vi "tcp_server_monitor.vi"(11 "TCP Socket Server in":refnum<data-value>) -> ()   [LabVIEW 2019, in "TCP Socket Server.lvclass"]
uses:
  TCP Socket Server.lvclass
  TCP Socket Server.lvclass/TCP Socket Server.ctl
  Utility API/Log Service/public/level.ctl
  df063e67-b3ba-41cf-b203-ca072a03e9e6.vi
  6658b09d-3cc9-4502-9e9e-f034e714faf1.vi
  e82c1857-569d-4e52-8d07-6a4305579ab7.vi
  Util/Timestamp or now.vi
  TCP Connection/TCP Connection.lvclass
  C:/Users/Nicholas Folse/Documents/workspace/github-tauterra.llc/ANODE/ANODE/Socket API/Connection/Connection.lvclass
  Socket Server/subVIs/spawn_connection_handler.vi
  Utility API/Log Service/Log Service.lvclass
  Socket Server/Socket Server.lvclass
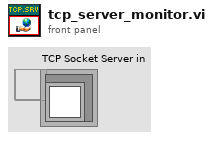
[diagram p1: front panel]
types:
  T1 = typedef "Utility API.lvlib/Log Service.lvclass/level.ctl" = u16
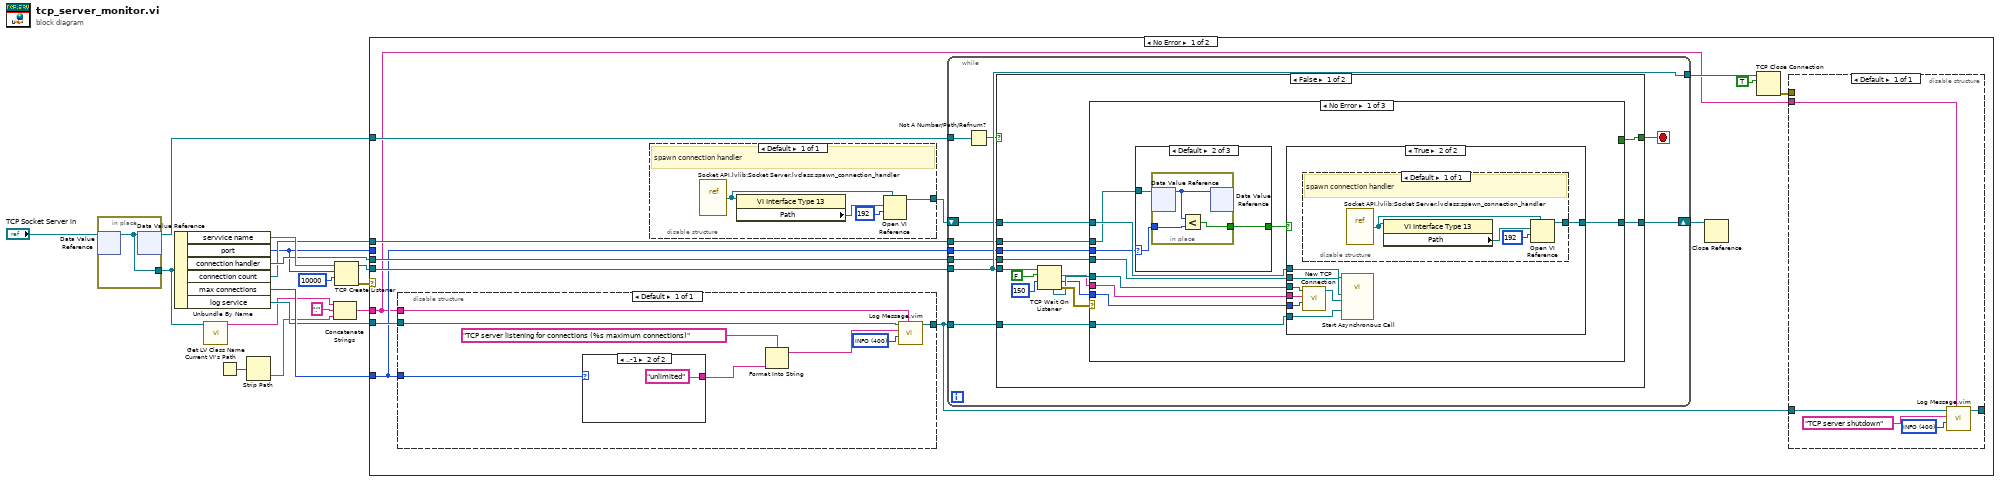
[diagram p0: block diagram]
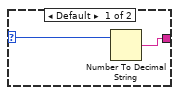
[diagram p2: hidden frame]
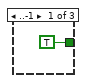
[diagram p3: hidden frame]
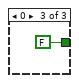
[diagram p4: hidden frame]
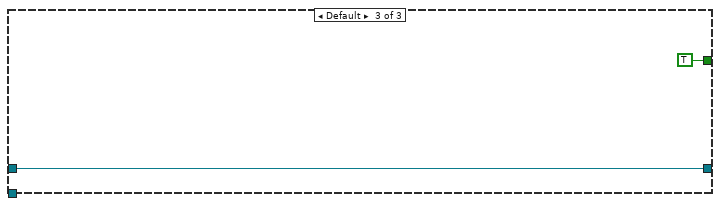
[diagram p7: hidden frame]
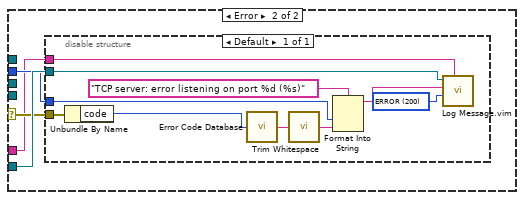
[diagram p9: hidden frame]
diagram:
  n1 = in-place {
    in-place-border: [w18] -> w5
    n2 = in-place-dvr #1("TCP Socket Server in") -> (w18:refnum<class "TCP Socket Server.lvclass">)  [unwired: 1 out]
    n3 = in-place-dvr #1(w18) -> (w11:refnum<data-value>)  [unwired: 1 out]
  }
  n4 = Unbundle By Name(w5) -> ("servvice name"=w16:string, "port"=w6:u16, "connection handler"=w12:refnum<class "Connection Handler.lvclass">, "connection count"=w10:refnum<data-value>, "max connections"=w9:i32, "log service"=w8:refnum<data-value>)
  n5 = call <vilib>:"Get LV Class Name.vi"("object"=w5) -> ("class name"=w3:string)  [unwired: 9 in, 1 out]
  n6 = Current VI's Path() -> (path=w7:path)
  n7 = Strip Path(path=w7) -> (name=w2:string)  [unwired: 1 out]
  n8 = Concatenate Strings(w3, ":" ("string"), w2) -> (w1:string)
  n9 = TCP Create Listener(9:10000 ("timeout ms (25000)"), 10:w6, 11:w16) -> (0:w14:errorcluster, 3:w13:refnum<k5>)  [unwired: 2 in, 1 out]
  n10 = case shown="No Error" w14 {
    selector: w14 -> [_ w114]
    tunnel: w13 -> [w31 _]
    tunnel: w11 -> [w30 _]
    tunnel: w12 -> [w27 _]
    tunnel: w10 -> [w24 _]
    tunnel: w9 -> [w22 _]
    tunnel: w8 -> [w23 w115]
    tunnel: w1 -> [w19 w112]
    tunnel: w6 -> [_ w113]
    frame No Error {
      n11 = disable-structure shown="Default" {
        disable-tunnel: w23 -> [w44]
        disable-tunnel: w22 -> [w43]
        disable-tunnel: w19 -> [w41]
        disable-tunnel: [w37] -> w20
        frame Enabled {
          w42 = T1 400 items=["OFF"=0, "FATAL"=100, "ERROR"=200, "WARN"=300, "INFO"=400, "DEBUG"=500, "TRACE"=600, "ALL"=65535] ("level")
          n12 = case shown="..-1" w43 {
            selector: w43 -> [w46 _]
            tunnel: [w45 "unlimited"] -> w39
            frame Default {
              n13 = Number To Decimal String(number=w46) -> (decimal integer string=w45:string)  [unwired: 1 in]
            }
            frame ..-1 {
            }
          }
          n14 = Format Into String(format string="TCP server listening for connections (%s maximum connections)" ("message"), w39) -> (resulting string=w38:string)  [unwired: 2 in, 1 out]
          n15 = call "Log Message.vim"("context"=w41, "level"=w42, "message"=w38, "Log Service in"=w44) -> ("Log Service out"=w37:refnum<data-value>)  [unwired: 6 in, 1 out]
        }
      }
      n16 = disable-structure shown="Default" {
        disable-tunnel: [w48] -> w26
        frame Enabled {
          # "spawn connection handler"
          n17 = vi-ref "Socket API.lvlib:Socket Server.lvclass:spawn_connection_handler.vi"() -> (w49:refnum<vi>)
          n18 = property class="VI Interface Type 13"(reference=w49) -> ("Path"=w50:path)  [unwired: 1 in, 2 out]
          n19 = Open VI Reference(type specifier VI Refnum (for type only)=w49, vi path=w50, options=192) -> (vi reference=w48:refnum<vi>)  [unwired: 3 in, 1 out]
        }
      }
      n20 = while {
        tunnel: w31 -> [w61]
        tunnel: w30 -> [w59]
        tunnel: [w61] -> w29
        tunnel: w27 -> [w60]
        shift-right: [w55] -> w25
        shift-left: w26 -> [w56]
        tunnel: w24 -> [w54]
        tunnel: w22 -> [w53]
        tunnel: w20 -> [w52]
        stop <- w57 stop-if-true
        n21 = Not A Number/Path/Refnum?(number/path/refnum=w59) -> (NaN/Path/Refnum?=w58:bool)
        n22 = case shown="False" w58 {
          selector: w58 -> [_ w111]
          tunnel: [w70 w111] -> w57
          tunnel: w61 -> [w75 _]
          tunnel: w60 -> [w67 _]
          tunnel: w56 -> [w66 w110]
          tunnel: [w65 w110] -> w55
          tunnel: w54 -> [w64 _]
          tunnel: w53 -> [w63 _]
          tunnel: w52 -> [w62 _]
          frame False {
            n23 = TCP Wait On Listener(9:150 ("timeout ms (wait forever: -1)"), 10:FALSE ("resolve remote address (T)"), 11:w75) -> (0:w72:errorcluster, 1:w68:u16, 2:w69:string, 4:w71:refnum<k5>)  [unwired: 1 in, 1 out]
            n24 = case shown="No Error" w72 {
              tunnel: w71 -> [w85 _ _]
              tunnel: [_ _ TRUE] -> w70
              tunnel: w69 -> [w84 _ _]
              tunnel: w68 -> [w83 _ _]
              tunnel: w67 -> [w82 _ _]
              tunnel: w66 -> [w81 w107 w108]
              tunnel: [w80 w107 w108] -> w65
              tunnel: w64 -> [w79 _ _]
              tunnel: w63 -> [w77 _ _]
              tunnel: w62 -> [w76 _ _]
              frame No Error {
                n25 = case shown="Default" w77 {
                  selector: w77 -> [_ w87 _]
                  tunnel: w79 -> [_ w89 _]
                  tunnel: [TRUE w88 FALSE] -> w78
                  frame ..-1 {
                  }
                  frame Default {
                    n26 = in-place {
                      in-place-border: w87 -> [w92]
                      in-place-border: [w90] -> w88
                      n27 = in-place-dvr #2(w89) -> (w91:i32)  [unwired: 1 out]
                      n28 = Less?(x=w91, y=w92) -> (x < y?=w90:bool)
                      n29 = in-place-dvr #2(w91) -> ()  [unwired: 2 out]
                    }
                  }
                  frame 0 {
                  }
                }
                n30 = case shown="True" w78 {
                  tunnel: w85 -> [_ w102]
                  tunnel: w84 -> [_ w101]
                  tunnel: w83 -> [_ w100]
                  tunnel: w82 -> [_ w99]
                  tunnel: w81 -> [w94 w97]
                  tunnel: [w94 w96] -> w80
                  tunnel: w76 -> [_ w95]
                  frame False {
                  }
                  frame True {
                    n31 = disable-structure shown="Default" {
                      disable-tunnel: [w103] -> w96
                      frame Enabled {
                        # "spawn connection handler"
                        n32 = vi-ref "Socket API.lvlib:Socket Server.lvclass:spawn_connection_handler.vi"() -> (w104:refnum<vi>)
                        n33 = property class="VI Interface Type 13"(reference=w104) -> ("Path"=w105:path)  [unwired: 1 in, 2 out]
                        n34 = Open VI Reference(type specifier VI Refnum (for type only)=w104, vi path=w105, options=192) -> (vi reference=w103:refnum<vi>)  [unwired: 3 in, 1 out]
                      }
                    }
                    n35 = call "New TCP Connection.vi"("remote port"=w100, "remote address"=w101, "connection ID"=w102) -> ("TCP Connection out"=w98:refnum<class "TCP Connection.lvclass">)  [unwired: 7 in, 1 out]
                    n36 = call-by-ref "Start Asynchronous Call"(reference=w97, "Log Service"=w95, "Connection"=w98, "Connection Hanlder"=w99) -> ()  [unwired: 10 in, 2 out]
                  }
                }
              }
              frame Error {
                # "timeout"
              }
              frame Default {
              }
            }
          }
          frame True {
          }
        }
      }
      n37 = Close Reference(reference=w25) -> ()  [unwired: 1 in, 1 out]
      n38 = TCP Close Connection(connection ID=w29, abort (F)=TRUE) -> (error out=w21:errorcluster)  [unwired: 1 in, 1 out]
      n39 = disable-structure shown="Default" {
        disable-tunnel: w20 -> [w36]
        disable-tunnel: w19 -> [w34]
        disable-tunnel: [w33] -> _
        disable-tunnel: w21 -> [_]
        frame Enabled {
          w35 = T1 400 items=["OFF"=0, "FATAL"=100, "ERROR"=200, "WARN"=300, "INFO"=400, "DEBUG"=500, "TRACE"=600, "ALL"=65535] ("level")
          n40 = call "Log Message.vim"("context"=w34, "level"=w35, "message"="TCP server shutdown", "Log Service in"=w36) -> ("Log Service out"=w33:refnum<data-value>)  [unwired: 6 in, 1 out]
        }
      }
    }
    frame Error {
      n41 = disable-structure shown="Default" {
        disable-tunnel: w115 -> [w125]
        disable-tunnel: w114 -> [w123]
        disable-tunnel: w113 -> [w120]
        disable-tunnel: w112 -> [w116]
        frame Enabled {
          w124 = T1 200 items=["OFF"=0, "FATAL"=100, "ERROR"=200, "WARN"=300, "INFO"=400, "DEBUG"=500, "TRACE"=600, "ALL"=65535] ("level")
          n42 = Unbundle By Name(w123) -> ("code"=w122:i32)
          n43 = call <vilib>:"Error Code Database.vi"("Error Code"=w122) -> ("Error Text"=w119:string)
          n44 = call <vilib>:"Trim Whitespace.vi"("string"=w119) -> ("trimmed string"=w118:string)  [unwired: 1 in]
          n45 = Format Into String(format string="TCP server: error listening on port %d (%s)" ("message"), w120, w118) -> (resulting string=w117:string)  [unwired: 2 in, 1 out]
          n46 = call "Log Message.vim"("context"=w116, "level"=w124, "message"=w117, "Log Service in"=w125) -> ()  [unwired: 6 in, 2 out]
        }
      }
    }
  }
